vi "Available White Position Read.vi"(4 "error in (no error)":errorcluster caption="错误输入（无错误）", 6 "Container State":T5 caption="容器状态", 7 "Display State In":T1={"method"=enum."None", "current color"=1, "available black position"=[], "available white position"=[], "Interactive Action"=refnum, "row"=0, "column"=0} caption="显示状态输入") -> (0 "error out":errorcluster caption="错误输出", 2 "Value":i32[][](array[numeric]), 3 "Display State Out":T1={"method"=enum."None", "current color"=1, "available black position"=[], "available white position"=[], "Interactive Action"=refnum, "row"=0, "column"=0} caption="显示状态输出")   [LabVIEW 2011, in "Othello.xctl"]
uses:
  Othello.xctl
  <vilib>/_xctls/Container State.ctl
  Ability/State.ctl
  Control/Method Call.ctl
  Control/Pict Ring Chess.ctl
  Control/Interactive Action.ctl
  <vilib>/_xctls/XControlSupport.lvlib
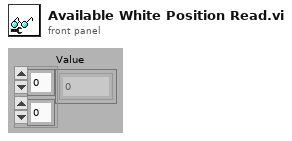
[diagram p1: front panel]
types:
  T1 = typedef "Othello.xctl/State.ctl" = cluster{"method":T2, "current color":T3, "available black position":i32[][], "available white position":i32[][], "Interactive Action":T4, "row":i32, "column":i32}
  T2 = typedef "Othello.xctl/Method Call.ctl" = enum16{"None", "New Game", "Play One"}
  T3 = typedef "Othello.xctl/Pict Ring Chess.ctl" = u16
  T4 = typedef "Othello.xctl/Interactive Action.ctl" = refnum<user-event>
  T5 = typedef "XControlSupport.lvlib/Container State.ctl" = cluster{"Indicator?":bool, "Run Mode?":bool, " Refnum":refnum<vi>}
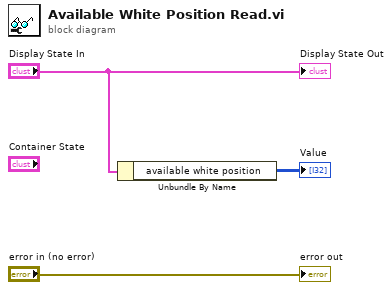
[diagram p0: block diagram]
diagram:
  n1 = Unbundle By Name("Display State In") -> ("available white position"=→"Value":i32[][])
  "error out" <- "error in (no error)"
  "Display State Out" <- "Display State In"
